vi "gRPC Client Test.vi"() -> ()   [LabVIEW 2024, in "pumploop_client.lvlib"]
uses:
  pumploop_client.lvlib
  controls/Controls--cluster.ctl
  controls/Sensors--cluster.ctl
  controls/SystemInfo--cluster.ctl
  controls/Valves--cluster.ctl
  <vilib>/gRPC/LabVIEW gRPC Library/Shared/grpcId.ctl
  controls/States.ctl
  controls/UI Queue Element.ctl
  RPC Messages/pumploop_GetSysInfRequest.ctl
  RPC Messages/pumploop_GetValveRequest.ctl
  RPC Messages/pumploop_GetControlRequest.ctl
  RPC Messages/pumploop_Controls.ctl
  RPC Messages/pumploop_Valves.ctl
  RPC Messages/pumploop_GetSensorRequest.ctl
  RPC Messages/pumploop_SystemInfo.ctl
  <vilib>/gRPC/LabVIEW gRPC Library/grpc-lvsupport-release.lvlib
panel:
  in  "Server Address":string="10.42.0.1:50051"
  in  "gRPC Disconnect":bool
  in  "gRPC Connect":bool
  in  "Stop":bool
  out "Error":errorcluster
  in  "Control Valves":T1
  out "Node Info":T2
  out "Sensors":T3 {"Pump Speed" scale=0.0..10.0; "Ambient Pressure" scale=0.5..1.5; "DUT Outlet Pressure" scale=0.0..2.0; "DUT Inlet Pressure" scale=0.0..10.0; "Flow" scale=0.0..100.0; "Sump Level" scale=0.0..100.0; "Tank Level" scale=0.0..100.0; "DUT Temp" scale=0.0..150.0; "Pump Temp" scale=0.0..150.0; "Tank Temp" scale=0.0..100.0; "Ambient Temp" scale=0.0..50.0}
  in  "Pump Control":T4
  in  "Stream":enum16{"Disabled", "Enabled"}(ring)
  in  "Subsystem":T5(ring)
  in  "Get/Set":enum16{"Get", "Set"}(ring)
  out "gRPC ID Out":u64
  # "192.168.0.141:50051"
  # "Open"
  # "Closed"
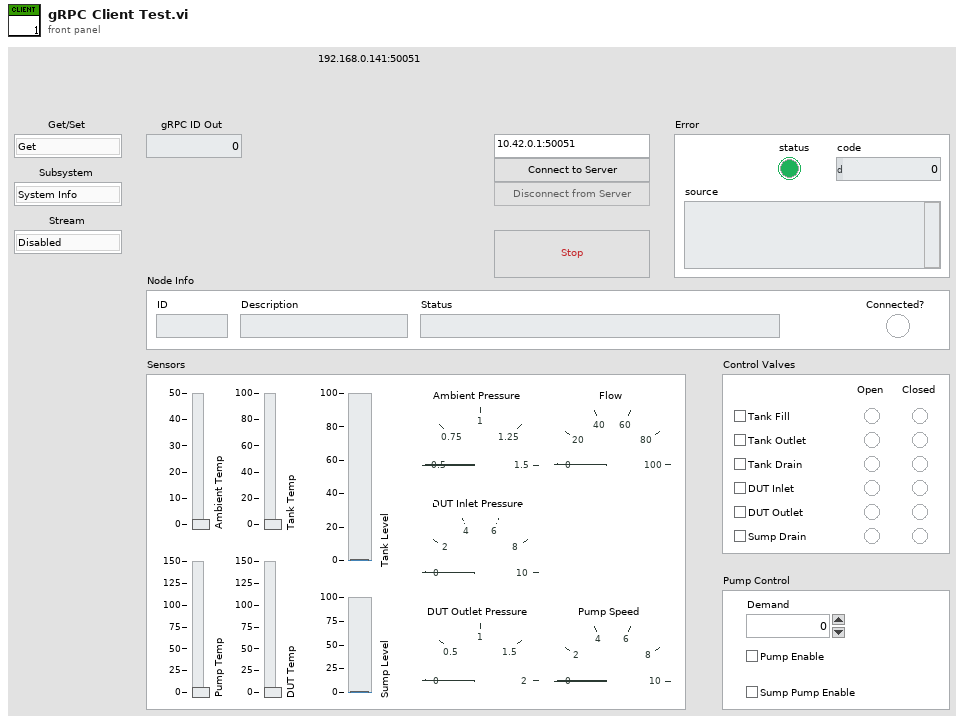
[diagram p1: front panel]
types:
  T1 = typedef "Valves--cluster.ctl" = cluster{"Tank Fill":bool, "Tank Outlet":bool, "Tank Drain":bool, "DUT Inlet":bool, "DUT Outlet":bool, "Sump Drain":bool, "Tank Fill Open":bool, "Tank Fill Closed":bool, "Tank Outlet Open":bool, "Tank Outlet Closed":bool, "Tank Drain Open":bool, "Tank Drain Closed":bool, "DUT Inlet Open":bool, "DUT Inlet Closed":bool, "DUT Outlet Open":bool, "DUT Outlet Closed":bool, "Sump Drain Open":bool, "Sump Drain Closed":bool}
  T2 = typedef "SystemInfo--cluster.ctl" = cluster{"Connected?":bool, "ID":string, "Description":string, "Status":string}
  T3 = typedef "Sensors--cluster.ctl" = cluster{"Tank Level":dbl, "Tank Temp":dbl, "Flow":dbl, "Pump Temp":dbl, "Pump Speed":dbl, "DUT Inlet Pressure":dbl, "DUT Outlet Pressure":dbl, "DUT Temp":dbl, "Sump Level":dbl, "Ambient Temp":dbl, "Ambient Pressure":dbl}
  T4 = typedef "Controls--cluster.ctl" = cluster{"Pump Enable":bool, "Demand":dbl, "Sump Pump Enable":bool}
  T5 = enum16{"System Info", "Valves", "Sensors", "Control"}
  T6 = typedef "UI Queue Element.ctl" = cluster{T7, variant}
  T7 = typedef "States.ctl" = enum16{"Initialise", "gRPC_Connect", "gRPC_Disconnect", "gRPC_Update-PumpCtrl", "gRPC_Update-ValveCtrl", "gRPC_ReadAll", "Update Settings", "Stop", "Quit"}
  T8 = cluster{"Node Info":T2, "Control Valves":T1, "Pump Control":T4, "Sensors":T3, "address":string}
  T9 = typedef "grpc-lvsupport-release.lvlib/grpcId.ctl" = u64
  T10 = typedef "pumploop_client.lvlib/pumploop_GetSysInfRequest.ctl" = cluster{"request":bool}
  T11 = typedef "pumploop_client.lvlib/pumploop_SystemInfo.ctl" = cluster{"nodeID":i32, "nodeDescription":string, "statusMsg":string}
  T12 = typedef "pumploop_client.lvlib/pumploop_GetValveRequest.ctl" = cluster{"request":bool}
  T13 = typedef "pumploop_client.lvlib/pumploop_Valves.ctl" = cluster{"tankFillIV":bool, "tankOutIV":bool, "tankDrainIV":bool, "dutInIV":bool, "dutOutIV":bool, "sumpDrainIV":bool}
  T14 = typedef "pumploop_client.lvlib/pumploop_GetSensorRequest.ctl" = cluster{"request":bool}
  T15 = typedef "pumploop_client.lvlib/pumploop_GetControlRequest.ctl" = cluster{"request":bool}
  T16 = typedef "pumploop_client.lvlib/pumploop_Controls.ctl" = cluster{"pumpEnable":bool, "pumpDemand":sgl, "sumppumpEnable":bool}
  T17 = typedef "pumploop_client.lvlib/pumploop_Sensors.ctl" = cluster{"tankLevel":sgl, "tankTemp":sgl, "dutFlow":sgl, "pumpTemp":sgl, "pumpSpeed":sgl, "dutPressIn":sgl, "dutPressOut":sgl, "dutTemp":sgl, "sumpLevel":sgl, "ambientTemp":sgl, "ambientPress":sgl}
  T18 = enum8{"Enabled", "Disabled", "Disabled and Grayed Out"}
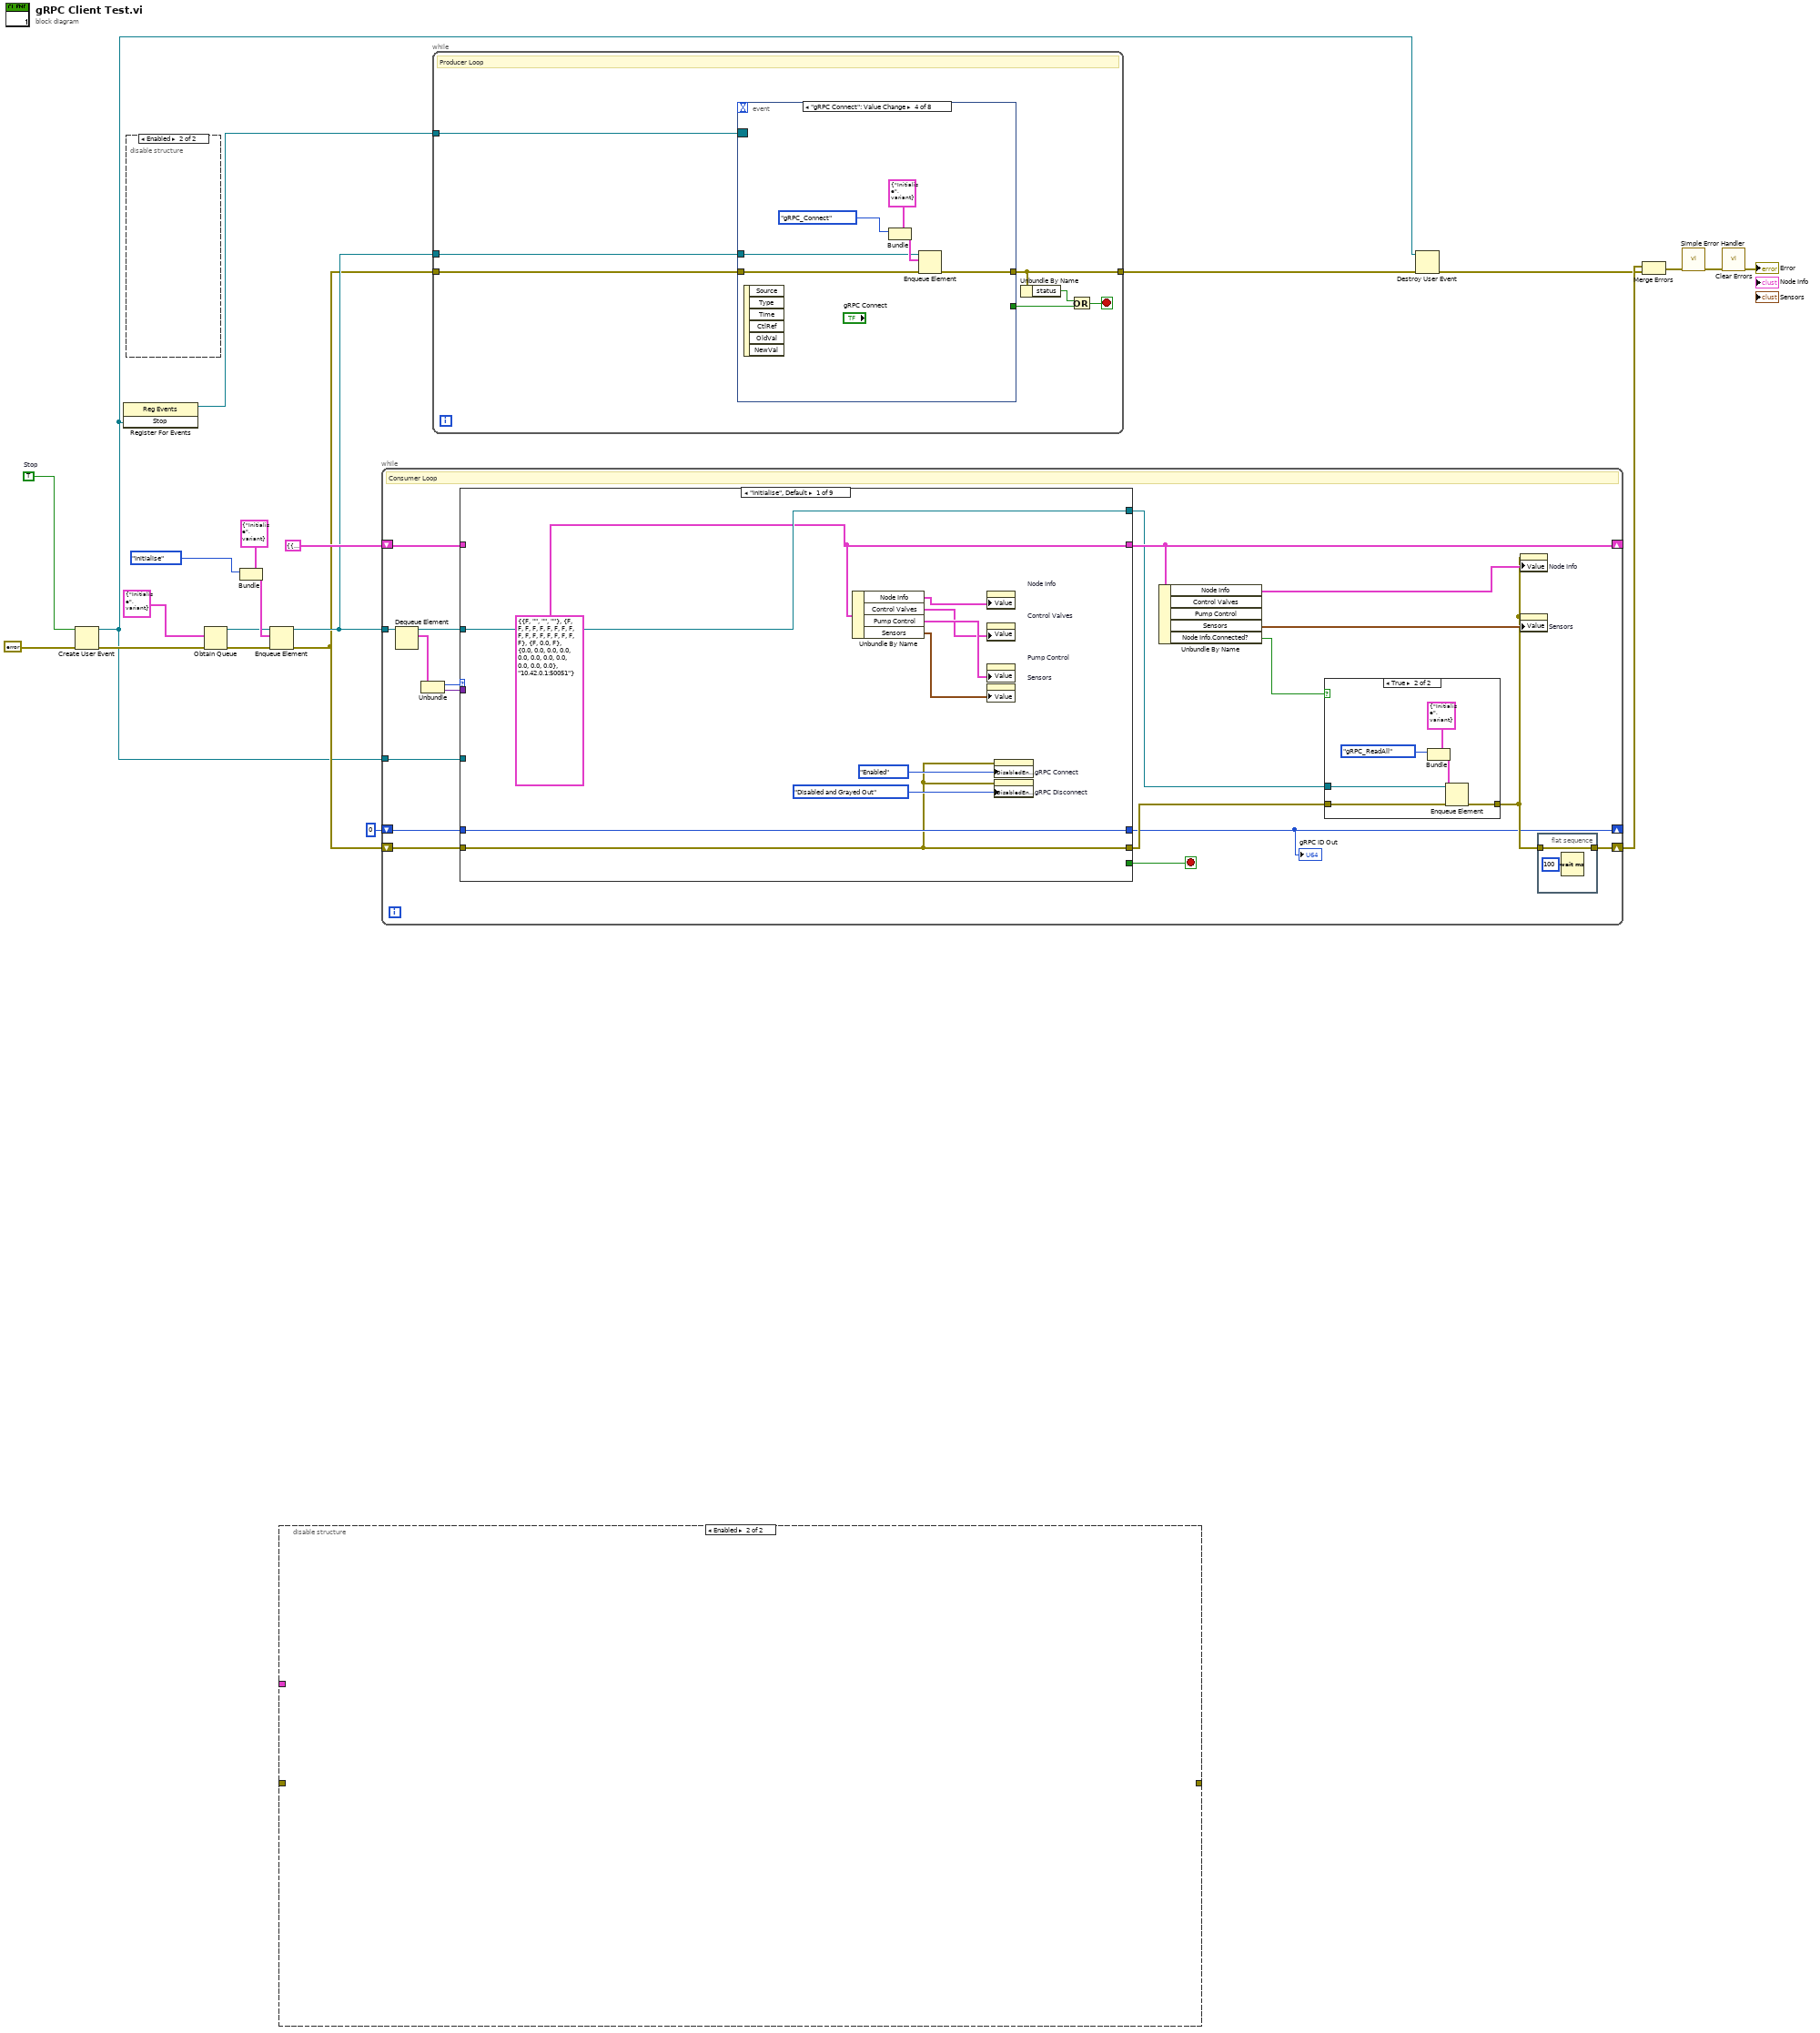
[diagram p0: block diagram]
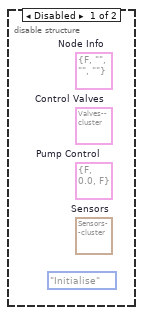
[diagram p2: hidden frame]
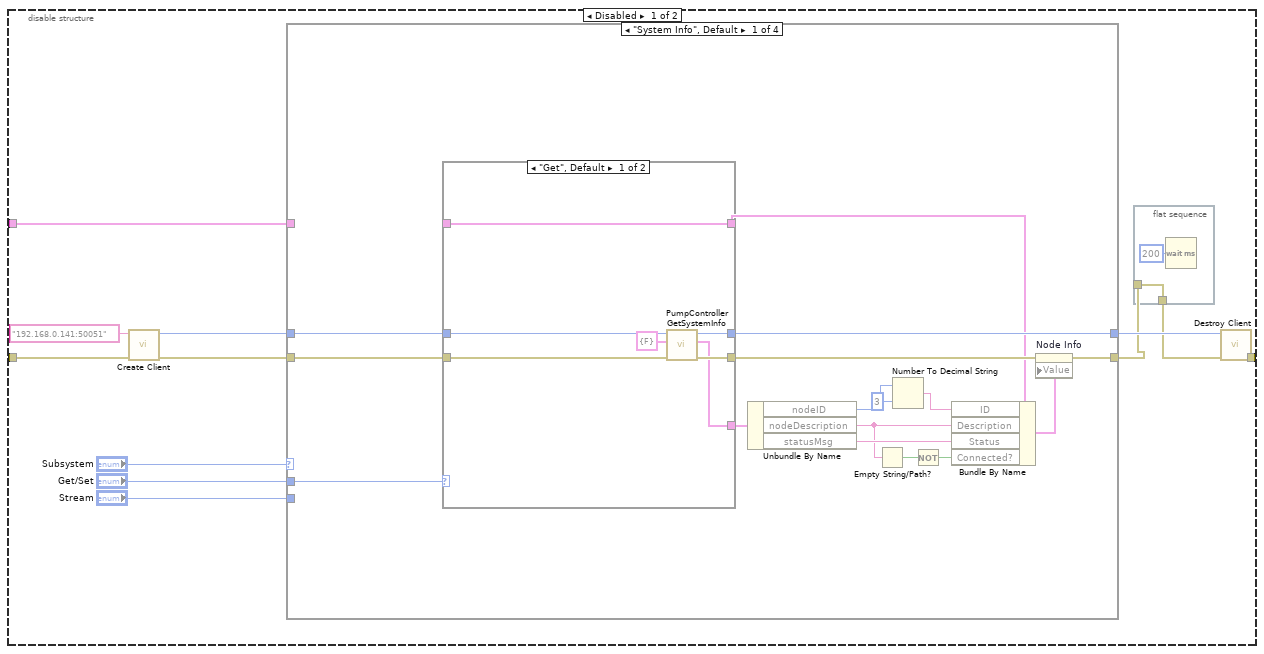
[diagram p3: hidden frame]
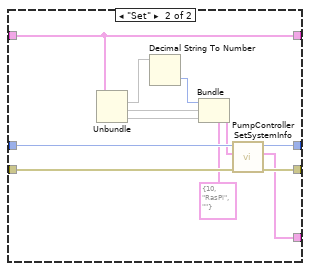
[diagram p4: hidden frame]
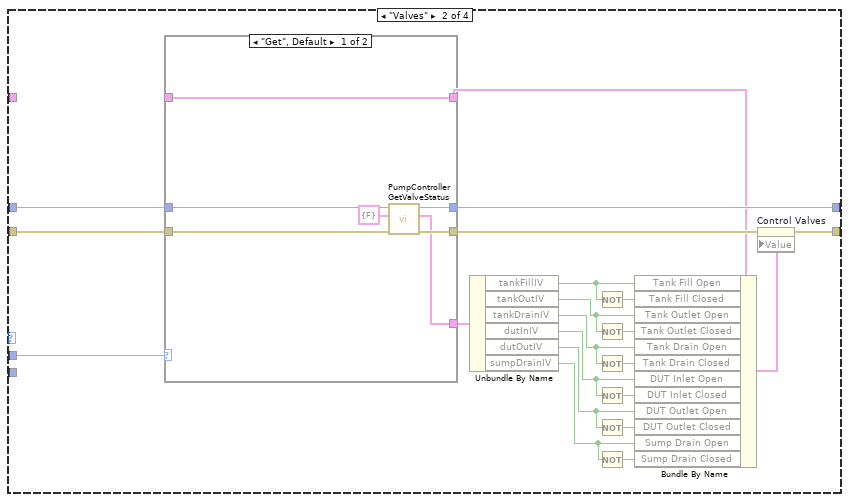
[diagram p5: hidden frame]
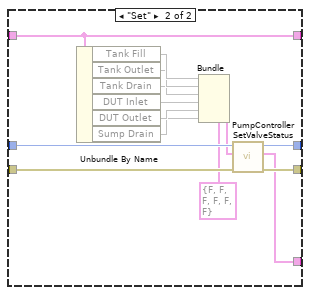
[diagram p6: hidden frame]
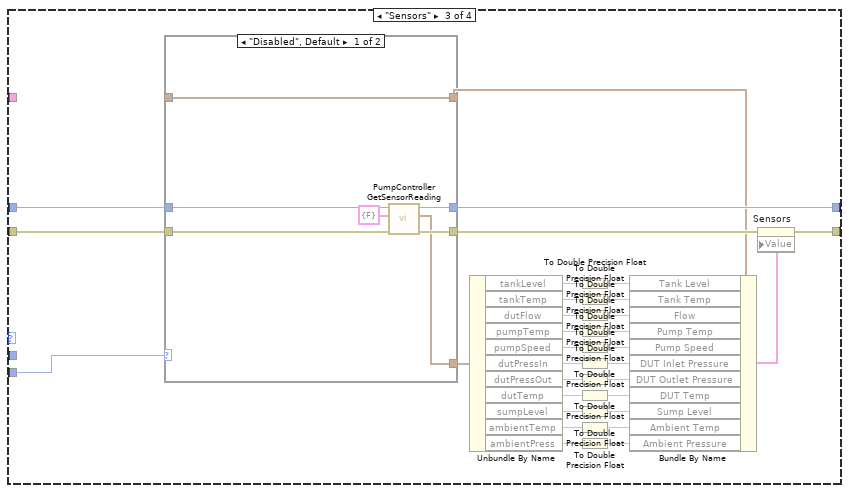
[diagram p7: hidden frame]
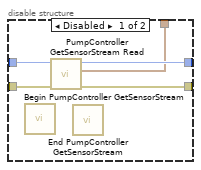
[diagram p9: hidden frame]
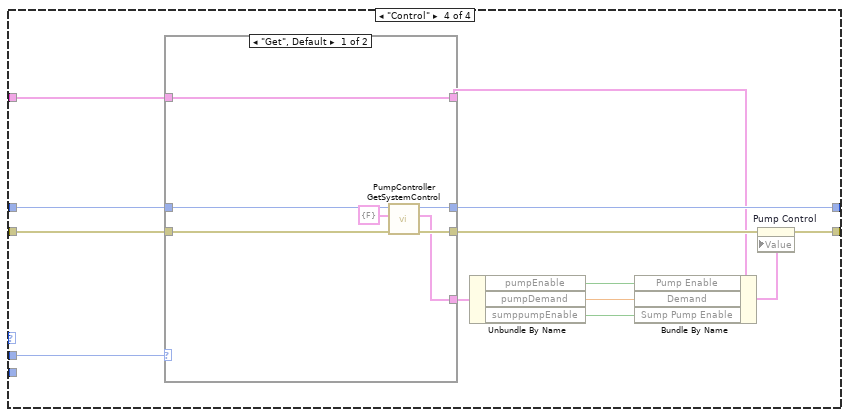
[diagram p10: hidden frame]
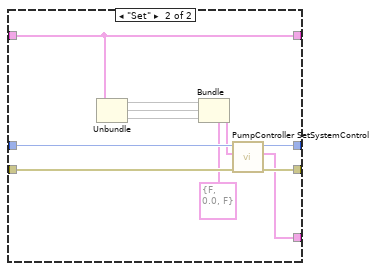
[diagram p11: hidden frame]
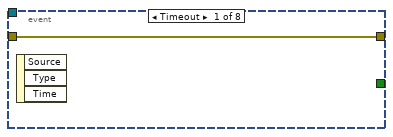
[diagram p12: hidden frame]
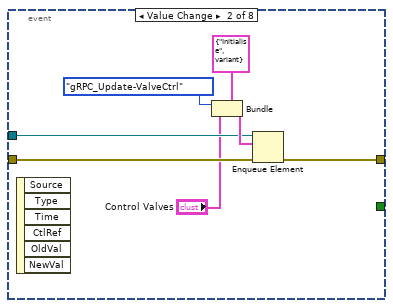
[diagram p13: hidden frame]
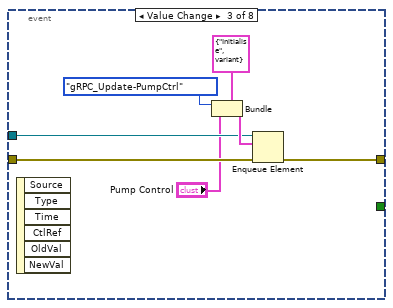
[diagram p14: hidden frame]
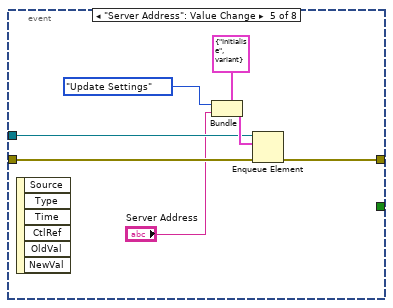
[diagram p15: hidden frame]
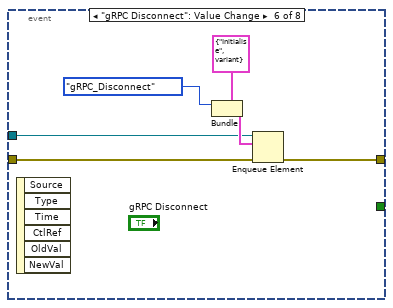
[diagram p16: hidden frame]
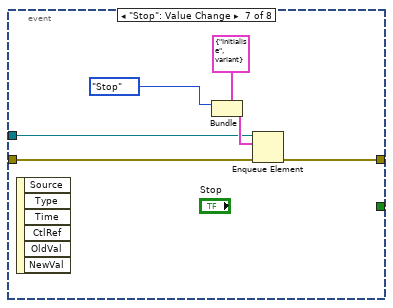
[diagram p17: hidden frame]
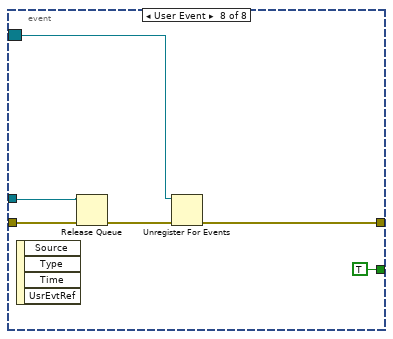
[diagram p18: hidden frame]
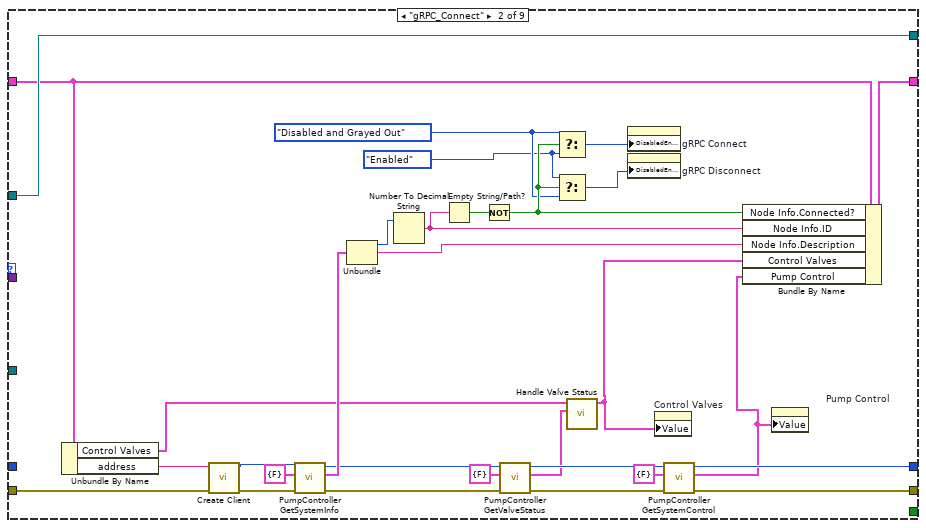
[diagram p20: hidden frame]
diagram:
  w7 = TRUE  # Stop
  n1 = Create User Event(user event datatype=w7, error in=errorcluster {"status"=FALSE, "code"=0, "source"=""}) -> (user event=w1:refnum<user-event>, error out=w5:errorcluster)
  n2 = register-events(w1) -> (reference out=w4:refnum<event-registration>)  [unwired: 2 in, 1 out]
  n3 = disable-structure shown="Enabled" {
    frame Disabled {
      (unwired) States."Initialise"
      (unwired) T3 {"Tank Level"=0.0, "Tank Temp"=0.0, "Flow"=0.0, "Pump Temp"=0.0, "Pump Speed"=0.0, "DUT Inlet Pressure"=0.0, "DUT Outlet Pressure"=0.0, "DUT Temp"=0.0, "Sump Level"=0.0, "Ambient Temp"=0.0, "Ambient Pressure"=0.0}  # Sensors
      (unwired) T4 {"Pump Enable"=FALSE, "Demand"=0.0, "Sump Pump Enable"=FALSE}  # Pump Control
      (unwired) T1 {"Tank Fill"=FALSE, "Tank Outlet"=FALSE, "Tank Drain"=FALSE, "DUT Inlet"=FALSE, "DUT Outlet"=FALSE, "Sump Drain"=FALSE, "Tank Fill Open"=FALSE, "Tank Fill Closed"=FALSE, "Tank Outlet Open"=FALSE, "Tank Outlet Closed"=FALSE, "Tank Drain Open"=FALSE, "Tank Drain Closed"=FALSE, "DUT Inlet Open"=FALSE, "DUT Inlet Closed"=FALSE, "DUT Outlet Open"=FALSE, "DUT Outlet Closed"=FALSE, "Sump Drain Open"=FALSE, "Sump Drain Closed"=FALSE}  # Control Valves
      (unwired) T2 {"Connected?"=FALSE, "ID"="", "Description"="", "Status"=""}  # Node Info
    }
    frame Enabled {
    }
  }
  n4 = Obtain Queue(element data type=T6 {enum."Initialise", variant}, error in (no error)=w5) -> (queue out=w12:refnum<queue>, error out=w11:errorcluster)  [unwired: 3 in, 1 out]
  n5 = Bundle(cluster=T6 {enum."Initialise", variant}, States."Initialise") -> (w15:T6)  [unwired: 1 in]
  n6 = Enqueue Element(queue=w12, element=w15, error in (no error)=w11) -> (queue out=w10:refnum<queue>, error out=w9:errorcluster)  [unwired: 1 in, 1 out]
  n7 = disable-structure shown="Enabled" {
    disable-tunnel: [w26 _] -> _
    disable-tunnel: _ -> [w23 _]
    disable-tunnel: _ -> [w22 _]
    frame Disabled {
      n8 = call "Create Client.vi"("error in"=w23, "address"="192.168.0.141:50051") -> ("error out"=w33:errorcluster, "gRPC ID Out"=w31:T9)  [unwired: 8 in]
      n9 = case shown="\"System Info\", Default" "Subsystem" {
        tunnel: w33 -> [w51 w91 w143 w174]
        tunnel: [w46 w87 w114 w166] -> w25
        tunnel: [w50 w90 w142 w173] -> w32
        tunnel: w31 -> [w49 w89 w141 w172]
        tunnel: "Get/Set" -> [w48 w88 _ w171]
        tunnel: "Stream" -> [_ _ w140 _]
        tunnel: w22 -> [_ _ _ w162]
        frame "System Info", Default {
          n10 = case shown="\"Get\", Default" w48 {
            tunnel: w51 -> [w58 w70]
            tunnel: [w56 w69] -> w47
            tunnel: [w55 w68] -> w50
            tunnel: w49 -> [w57 w67]
            tunnel: [w54 w66] -> w45
            tunnel: _ -> [w52 w64]
            tunnel: [w52 w64] -> w39
            frame "Get", Default {
              n11 = call "PumpController GetSystemInfo.vi"("error in"=w58, "Request Data"=T10 {"request"=FALSE}, "gRPC ID"=w57) -> ("error out"=w56:errorcluster, "Response Data"=w54:T11, "gRPC ID out"=w55:T9)  [unwired: 6 in]
            }
            frame "Set" {
              n12 = Unbundle(w64) -> ("ID"=w60, "Description"=w62, "Status"=w61)  [unwired: 1 out]
              n13 = Decimal String To Number(string=w60) -> (number=w59:i32)  [unwired: 2 in, 1 out]
              n14 = Bundle(cluster=T11 {"nodeID"=10, "nodeDescription"="RasPi", "statusMsg"=""} ("Node Info Request"), "nodeID"=w59, "nodeDescription"=w62, "statusMsg"=w61) -> (w63:T11)
              n15 = call "PumpController SetSystemInfo.vi"("error in"=w70, "Request Data"=w63, "gRPC ID"=w67) -> ("error out"=w69:errorcluster, "Response Data"=w66:T11, "gRPC ID out"=w68:T9)  [unwired: 6 in]
            }
          }
          n16 = Unbundle By Name(w45) -> ("nodeID"=w42:i32, "nodeDescription"=w38:string, "statusMsg"=w43:string)
          n17 = Empty String/Path?(string/path=w38) -> (empty?=w37:bool)
          n18 = Number To Decimal String(number=w42, width (-)=i16 3) -> (decimal integer string=w41:string)
          n19 = Not(x=w37) -> (.not. x?=w36:bool)
          n20 = Bundle By Name(cluster=w39, "ID"=w41, "Description"=w38, "Status"=w43, "Connected?"=w36) -> (w44:cluster{})
          n21 = property on="Node Info" class="Clust (strict)"(error in=w47, "Value"=w44) -> (error out=w46:errorcluster)  [unwired: 1 in, 1 out]
        }
        frame "Valves" {
          n22 = case shown="\"Get\", Default" w88 {
            tunnel: w91 -> [w97 w111]
            tunnel: [w96 w109] -> w86
            tunnel: [w95 w110] -> w90
            tunnel: w89 -> [w98 w112]
            tunnel: [w94 w108] -> w85
            tunnel: _ -> [w92 w99]
            tunnel: [w92 w99] -> w71
            frame "Get", Default {
              n23 = call "PumpController GetValveStatus.vi"("error in"=w97, "Request Data"=T12 {"request"=FALSE}, "gRPC ID"=w98) -> ("error out"=w96:errorcluster, "Response Data"=w94:T13, "gRPC ID out"=w95:T9)  [unwired: 6 in]
            }
            frame "Set" {
              n24 = Unbundle By Name(w99) -> ("Tank Fill"=w106, "Tank Outlet"=w105, "Tank Drain"=w104, "DUT Inlet"=w103, "DUT Outlet"=w102, "Sump Drain"=w101)
              n25 = Bundle(cluster=T13 {"tankFillIV"=FALSE, "tankOutIV"=FALSE, "tankDrainIV"=FALSE, "dutInIV"=FALSE, "dutOutIV"=FALSE, "sumpDrainIV"=FALSE} ("Valve Control Request"), "tankFillIV"=w106, "tankOutIV"=w105, "tankDrainIV"=w104, "dutInIV"=w103, "dutOutIV"=w102, "sumpDrainIV"=w101) -> (w100:T13)
              n26 = call "PumpController SetValveStatus.vi"("error in"=w111, "Request Data"=w100, "gRPC ID"=w112) -> ("error out"=w109:errorcluster, "Response Data"=w108:T13, "gRPC ID out"=w110:T9)  [unwired: 6 in]
            }
          }
          n27 = Unbundle By Name(w85) -> ("tankFillIV"=w76:bool, "tankOutIV"=w75:bool, "tankDrainIV"=w77:bool, "dutInIV"=w74:bool, "dutOutIV"=w73:bool, "sumpDrainIV"=w72:bool)
          n28 = Not(x=w76) -> (.not. x?=w83:bool)
          n29 = Not(x=w75) -> (.not. x?=w82:bool)
          n30 = Not(x=w77) -> (.not. x?=w81:bool)
          n31 = Not(x=w74) -> (.not. x?=w80:bool)
          n32 = Not(x=w73) -> (.not. x?=w79:bool)
          n33 = Not(x=w72) -> (.not. x?=w78:bool)
          n34 = Bundle By Name(cluster=w71, "Tank Fill Open"=w76, "Tank Fill Closed"=w83, "Tank Outlet Open"=w75, "Tank Outlet Closed"=w82, "Tank Drain Open"=w77, "Tank Drain Closed"=w81, "DUT Inlet Open"=w74, "DUT Inlet Closed"=w80, "DUT Outlet Open"=w73, "DUT Outlet Closed"=w79, "Sump Drain Open"=w72, "Sump Drain Closed"=w78) -> (w84:cluster{})
          n35 = property on="Control Valves" class="Clust (strict)"(error in=w86, "Value"=w84) -> (error out=w87:errorcluster)  [unwired: 1 in, 1 out]
        }
        frame "Sensors" {
          n36 = case shown="\"Disabled\", Default" w140 {
            tunnel: w143 -> [w147 w153]
            tunnel: [w149 w156] -> w115
            tunnel: [w150 w155] -> w142
            tunnel: w141 -> [w148 w154]
            tunnel: [w145 w152] -> w139
            tunnel: [w144 w151] -> w113
            tunnel: _ -> [w144 w151]
            frame "Disabled", Default {
              n37 = call "PumpController GetSensorReading.vi"("error in"=w147, "Request Data"=T14 {"request"=FALSE}, "gRPC ID"=w148) -> ("error out"=w149:errorcluster, "Response Data"=w145:T17, "gRPC ID out"=w150:T9)  [unwired: 6 in]
            }
            frame "Enabled" {
              n38 = disable-structure shown="Enabled" {
                disable-tunnel: [w161 _] -> w156
                disable-tunnel: [w160 _] -> w155
                disable-tunnel: w154 -> [w159 _]
                disable-tunnel: w153 -> [w158 _]
                disable-tunnel: [w157 _] -> w152
                frame Disabled {
                  n39 = call "Begin PumpController GetSensorStream.vi"() -> ()  [unwired: 9 in, 3 out]
                  n40 = call "PumpController GetSensorStream Read.vi"("error in"=w158, "Call ID in"=w159) -> ("error out"=w161:errorcluster, "Response Data"=w157:T17, "Call ID"=w160:T9)  [unwired: 6 in, 1 out]
                  n41 = call "End PumpController GetSensorStream.vi"() -> ()  [unwired: 10 in, 2 out]
                }
                frame Enabled {
                }
              }
            }
          }
          n42 = Unbundle By Name(w139) -> ("tankLevel"=w138:sgl, "tankTemp"=w137:sgl, "dutFlow"=w136:sgl, "pumpTemp"=w134:sgl, "pumpSpeed"=w133:sgl, "dutPressIn"=w135:sgl, "dutPressOut"=w132:sgl, "dutTemp"=w131:sgl, "sumpLevel"=w130:sgl, "ambientTemp"=w129:sgl, "ambientPress"=w128:sgl)
          n43 = To Double Precision Float(number=w138) -> (double precision float=w127:dbl)
          n44 = To Double Precision Float(number=w137) -> (double precision float=w126:dbl)
          n45 = To Double Precision Float(number=w136) -> (double precision float=w125:dbl)
          n46 = To Double Precision Float(number=w134) -> (double precision float=w124:dbl)
          n47 = To Double Precision Float(number=w133) -> (double precision float=w123:dbl)
          n48 = To Double Precision Float(number=w135) -> (double precision float=w122:dbl)
          n49 = To Double Precision Float(number=w132) -> (double precision float=w121:dbl)
          n50 = To Double Precision Float(number=w131) -> (double precision float=w120:dbl)
          n51 = To Double Precision Float(number=w130) -> (double precision float=w119:dbl)
          n52 = To Double Precision Float(number=w129) -> (double precision float=w118:dbl)
          n53 = To Double Precision Float(number=w128) -> (double precision float=w117:dbl)
          n54 = Bundle By Name(cluster=w113, "Tank Level"=w127, "Tank Temp"=w126, "Flow"=w125, "Pump Temp"=w124, "Pump Speed"=w123, "DUT Inlet Pressure"=w122, "DUT Outlet Pressure"=w121, "DUT Temp"=w120, "Sump Level"=w119, "Ambient Temp"=w118, "Ambient Pressure"=w117) -> (w116:cluster{})
          n55 = property on="Sensors" class="Clust (strict)"(error in=w115, "Value"=w116) -> (error out=w114:errorcluster)  [unwired: 1 in, 1 out]
        }
        frame "Control" {
          n56 = case shown="\"Get\", Default" w171 {
            tunnel: w174 -> [w180 w191]
            tunnel: [w178 w189] -> w165
            tunnel: [w179 w190] -> w173
            tunnel: w172 -> [w181 w192]
            tunnel: [w177 w188] -> w170
            tunnel: w162 -> [w175 w183]
            tunnel: [w175 w183] -> w163
            frame "Get", Default {
              n57 = call "PumpController GetSystemControl.vi"("error in"=w180, "Request Data"=T15 {"request"=FALSE}, "gRPC ID"=w181) -> ("error out"=w178:errorcluster, "Response Data"=w177:T16, "gRPC ID out"=w179:T9)  [unwired: 6 in]
            }
            frame "Set" {
              n58 = Unbundle(w183) -> ("Pump Enable"=w186, "Demand"=w187, "Sump Pump Enable"=w182)
              n59 = Bundle(cluster=T16 {"pumpEnable"=FALSE, "pumpDemand"=0.0, "sumppumpEnable"=FALSE} ("System Control Request"), "pumpEnable"=w186, "pumpDemand"=w187, "sumppumpEnable"=w182) -> (w185:T16)
              n60 = call "PumpController SetSystemControl.vi"("error in"=w191, "Request Data"=w185, "gRPC ID"=w192) -> ("error out"=w189:errorcluster, "Response Data"=w188:T16, "gRPC ID out"=w190:T9)  [unwired: 6 in]
            }
          }
          n61 = Unbundle By Name(w170) -> ("pumpEnable"=w169:bool, "pumpDemand"=w168:sgl, "sumppumpEnable"=w167:bool)
          n62 = Bundle By Name(cluster=w163, "Pump Enable"=w169, "Demand"=w168, "Sump Pump Enable"=w167) -> (w164:cluster{})
          n63 = property on="Pump Control" class="Clust (strict)"(error in=w165, "Value"=w164) -> (error out=w166:errorcluster)  [unwired: 1 in, 1 out]
        }
      }
      n64 = flat-sequence {
        tunnel: w25 -> [w35]
        tunnel: [w35] -> w24
        frame #0 {
          n65 = Wait (ms)(milliseconds to wait=u32 200) -> ()  [unwired: 1 out]
        }
      }
      n66 = call "Destroy Client.vi"("error in"=w24, "gRPC ID"=w32) -> ("error out"=w26:errorcluster)  [unwired: 9 in]
    }
    frame Enabled {
    }
  }
  n67 = while {
    shift-right: [w197] -> w18
    shift-left: w9 -> [w211]
    shift-right: [w194] -> _
    shift-left: T9 0 ("gRPC ID Out") -> [w210]
    tunnel: w10 -> [w209]
    shift-right: [w203] -> _
    shift-left: T8 {"Node Info"={"Connected?"=FALSE, "ID"="", "Description"="", "Status"=""}, "Control Valves"={"Tank Fill"=FALSE, "Tank Outlet"=FALSE, "Tank Drain"=FALSE, "DUT Inlet"=FALSE, "DUT Outlet"=FALSE, "Sump Drain"=FALSE, "Tank Fill Open"=FALSE, "Tank Fill Closed"=FALSE, "Tank Outlet Open"=FALSE, "Tank Outlet Closed"=FALSE, "Tank Drain Open"=FALSE, "Tank Drain Closed"=FALSE, "DUT Inlet Open"=FALSE, "DUT Inlet Closed"=FALSE, "DUT Outlet Open"=FALSE, "DUT Outlet Closed"=FALSE, "Sump Drain Open"=FALSE, "Sump Drain Closed"=FALSE}, "Pump Control"={"Pump Enable"=FALSE, "Demand"=0.0, "Sump Pump Enable"=FALSE}, "Sensors"={"Tank Level"=0.0, "Tank Temp"=0.0, "Flow"=0.0, "Pump Temp"=0.0, "Pump Speed"=0.0, "DUT Inlet Pressure"=0.0, "DUT Outlet Pressure"=0.0, "DUT Temp"=0.0, "Sump Level"=0.0, "Ambient Temp"=0.0, "Ambient Pressure"=0.0}, "address"="192.168.0.141:50051"} -> [w204]
    tunnel: w1 -> [w193]
    stop <- w200 stop-if-true
    # "Consumer Loop"
    n68 = Dequeue Element(queue=w209) -> (queue out=w206:refnum<queue>, element=w208:T6)  [unwired: 2 in, 2 out]
    n69 = Unbundle(w208) -> (w207:T7, w205:variant)
    n70 = case shown="\"Initialise\", Default" w207 {
      tunnel: w211 -> [w226 w260 w271 w277 w295 w299 w309 w339 w375]
      tunnel: [w226 w240 w263 w276 w287 w298 w312 w336 w374] -> w196
      tunnel: [w230 w237 T9 0 ("gRPC ID Out") w284 w286 w304 w311 w335 w373] -> w194
      tunnel: w210 -> [w230 _ w270 w284 w286 w304 w313 w337 w372]
      tunnel: w206 -> [w229 w259 w268 w283 w290 w301 w307 w334 w370]
      tunnel: w205 -> [_ _ _ w280 _ _ w310 w340 _]
      tunnel: w204 -> [_ w253 w261 w282 w285 w303 w306 w332 w369]
      tunnel: [w221 w252 w267 w281 w285 w303 w308 w338 w371] -> w203
      tunnel: [_ _ _ _ _ TRUE _ _ _] -> w200
      tunnel: [w229 w259 w268 w283 w290 w301 w307 w334 w370] -> w199
      tunnel: w193 -> [_ _ _ _ _ w300 _ _ _]
      frame "Initialise", Default {
        w221 = T8 {"Node Info"={"Connected?"=FALSE, "ID"="", "Description"="", "Status"=""}, "Control Valves"={"Tank Fill"=FALSE, "Tank Outlet"=FALSE, "Tank Drain"=FALSE, "DUT Inlet"=FALSE, "DUT Outlet"=FALSE, "Sump Drain"=FALSE, "Tank Fill Open"=FALSE, "Tank Fill Closed"=FALSE, "Tank Outlet Open"=FALSE, "Tank Outlet Closed"=FALSE, "Tank Drain Open"=FALSE, "Tank Drain Closed"=FALSE, "DUT Inlet Open"=FALSE, "DUT Inlet Closed"=FALSE, "DUT Outlet Open"=FALSE, "DUT Outlet Closed"=FALSE, "Sump Drain Open"=FALSE, "Sump Drain Closed"=FALSE}, "Pump Control"={"Pump Enable"=FALSE, "Demand"=0.0, "Sump Pump Enable"=FALSE}, "Sensors"={"Tank Level"=0.0, "Tank Temp"=0.0, "Flow"=0.0, "Pump Temp"=0.0, "Pump Speed"=0.0, "DUT Inlet Pressure"=0.0, "DUT Outlet Pressure"=0.0, "DUT Temp"=0.0, "Sump Level"=0.0, "Ambient Temp"=0.0, "Ambient Pressure"=0.0}, "address"="10.42.0.1:50051"}
        n71 = Unbundle By Name(w221) -> ("Node Info"=w223:T2, "Control Valves"=w222:T1, "Pump Control"=w224:T4, "Sensors"=w225:T3)
        n72 = property on="Node Info" class="Clust (strict)"("Value"=w223) -> ()  [unwired: 2 in, 2 out]
        n73 = property on="Control Valves" class="Clust (strict)"("Value"=w222) -> ()  [unwired: 2 in, 2 out]
        n74 = property on="Pump Control" class="Clust (strict)"("Value"=w224) -> ()  [unwired: 2 in, 2 out]
        n75 = property on="Sensors" class="Clust (strict)"("Value"=w225) -> ()  [unwired: 2 in, 2 out]
        n76 = property on="gRPC Connect" class="Bool (strict)"(error in=w226, "DisabledEnum"=T18."Enabled" ("Disabled")) -> ()  [unwired: 1 in, 2 out]
        n77 = property on="gRPC Disconnect" class="Bool (strict)"(error in=w226, "DisabledEnum"=T18."Disabled and Grayed Out" ("Disabled")) -> ()  [unwired: 1 in, 2 out]
      }
      frame "gRPC_Connect" {
        w245 = T18."Enabled" ("Disabled")
        w246 = T18."Disabled and Grayed Out" ("Disabled")
        n78 = Unbundle By Name(w253) -> ("Control Valves"=w233:T1, "address"=w258:string)
        n79 = call "Create Client.vi"("error in"=w260, "address"=w258) -> ("error out"=w250:errorcluster, "gRPC ID Out"=w249:T9)  [unwired: 8 in]
        n80 = call "PumpController GetSystemInfo.vi"("error in"=w250, "Request Data"=T10 {"request"=FALSE}, "gRPC ID"=w249) -> ("error out"=w241:errorcluster, "Response Data"=w254:T11, "gRPC ID out"=w239:T9)  [unwired: 6 in]
        n81 = Unbundle(w254) -> ("nodeID"=w257:i32, "nodeDescription"=w256:string)  [unwired: 1 out]
        n82 = Number To Decimal String(number=w257) -> (decimal integer string=w255:string)  [unwired: 1 in]
        n83 = Empty String/Path?(string/path=w255) -> (empty?=w248:bool)
        n84 = Not(x=w248) -> (.not. x?=w247:bool)
        n85 = call "PumpController GetValveStatus.vi"("error in"=w241, "Request Data"=T12 {"request"=FALSE}, "gRPC ID"=w239) -> ("error out"=w242:errorcluster, "Response Data"=w234:T13, "gRPC ID out"=w238:T9)  [unwired: 6 in]
        n86 = Select(t=w246, s=w247, f=w245) -> (s? t:f=w244:T18)
        n87 = Select(t=w245, s=w247, f=w246) -> (s? t:f=w243:T18)
        n88 = call "Handle Valve Status.vi"("Response Data"=w234, "Control Valves in"=w233) -> ("Control Valves out"=w232:T1)  [unwired: 9 in]
        n89 = property on="gRPC Connect" class="Bool (strict)"("DisabledEnum"=w244) -> ()  [unwired: 2 in, 2 out]
        n90 = property on="gRPC Disconnect" class="Bool (strict)"("DisabledEnum"=w243) -> ()  [unwired: 2 in, 2 out]
        n91 = property on="Control Valves" class="Clust (strict)"("Value"=w232) -> ()  [unwired: 2 in, 2 out]
        n92 = call "PumpController GetSystemControl.vi"("error in"=w242, "Request Data"=T15 {"request"=FALSE}, "gRPC ID"=w238) -> ("error out"=w240:errorcluster, "Response Data"=w231:T16, "gRPC ID out"=w237:T9)  [unwired: 6 in]
        n93 = Bundle By Name(cluster=w253, "Node Info.Connected?"=w247, "Node Info.ID"=w255, "Node Info.Description"=w256, "Control Valves"=w232, "Pump Control"=w231) -> (w252:T8)
        n94 = property on="Pump Control" class="Clust (strict)"("Value"=w231) -> ()  [unwired: 2 in, 2 out]
      }
      frame "gRPC_Disconnect" {
        n95 = Unbundle By Name(w261) -> ("Node Info.Connected?"=w262:bool)
        n96 = case shown="False" w262 {
          tunnel: w271 -> [w272 w275]
          tunnel: w270 -> [_ w274]
          tunnel: [w272 w273] -> w263
          frame False {
          }
          frame True {
            n97 = call "Destroy Client.vi"("error in"=w275, "gRPC ID"=w274) -> ("error out"=w273:errorcluster)  [unwired: 9 in]
          }
        }
        n98 = Bundle By Name(cluster=w261, "Node Info.Connected?"=FALSE) -> (w267:T8)
        n99 = property on="gRPC Connect" class="Bool (strict)"(error in=w263, "DisabledEnum"=T18."Enabled" ("Disabled")) -> ()  [unwired: 1 in, 2 out]
        n100 = property on="gRPC Disconnect" class="Bool (strict)"(error in=w263, "DisabledEnum"=T18."Disabled and Grayed Out" ("Disabled")) -> ()  [unwired: 1 in, 2 out]
      }
      frame "Update Settings" {
        n101 = Variant To Data(error in=w277, type="", Variant=w280) -> (data=w278:string, error out=w276:errorcluster)
        n102 = Bundle By Name(cluster=w282, "address"=w278) -> (w281:T8)
      }
      frame "Stop" {
        w288 = T6 {enum."Initialise", variant}
        n103 = Bundle(cluster=w288, States."gRPC_Disconnect") -> (w294:T6)  [unwired: 1 in]
        n104 = Enqueue Element(queue=w290, element=w294, error in (no error)=w295) -> (queue out=w291:refnum<queue>, error out=w292:errorcluster)  [unwired: 1 in, 1 out]
        n105 = Bundle(cluster=w288, States."Quit") -> (w289:T6)  [unwired: 1 in]
        n106 = Enqueue Element(queue=w291, element=w289, error in (no error)=w292) -> (error out=w287:errorcluster)  [unwired: 1 in, 2 out]
      }
      frame "Quit" {
        n107 = Generate User Event(user event=w300, event data cluster=TRUE ("event data"), error in=w299) -> (error out=w298:errorcluster)  [unwired: 1 in, 1 out]
      }
      frame "gRPC_Update-PumpCtrl" {
        n108 = Unbundle By Name(w306) -> ("Node Info.Connected?"=w305:bool)
        n109 = case shown="False" w305 {
          tunnel: w313 -> [w315 w326]
          tunnel: [w314 w325] -> w312
          tunnel: [w315 w324] -> w311
          tunnel: w310 -> [_ w323]
          tunnel: w309 -> [w314 w322]
          tunnel: w306 -> [w316 w319]
          tunnel: [w316 w317] -> w308
          frame False {
          }
          frame True {
            n110 = Variant To Data(error in=w322, type=T4 {"Pump Enable"=FALSE, "Demand"=0.0, "Sump Pump Enable"=FALSE} ("Pump Control"), Variant=w323) -> (data=w318:T4, error out=w321:errorcluster)
            n111 = Unbundle(w318) -> ("Pump Enable"=w328:bool, "Demand"=w327:dbl, "Sump Pump Enable"=w331:bool)
            n112 = Bundle(cluster=T16 {"pumpEnable"=FALSE, "pumpDemand"=0.0, "sumppumpEnable"=FALSE} ("System Control Request"), "pumpEnable"=w328, "pumpDemand"=w327, "sumppumpEnable"=w331) -> (w329:T16)
            n113 = Bundle By Name(cluster=w319, "Pump Control"=w318) -> (w317:T8)
            n114 = call "PumpController SetSystemControl.vi"("error in"=w321, "Request Data"=w329, "gRPC ID"=w326) -> ("error out"=w325:errorcluster, "gRPC ID out"=w324:T9)  [unwired: 6 in, 1 out]
          }
        }
      }
      frame "gRPC_Update-ValveCtrl" {
        n115 = Unbundle By Name(w332) -> ("Node Info.Connected?"=w333:bool)
        n116 = case shown="True" w333 {
          tunnel: w340 -> [_ w365]
          tunnel: w339 -> [w341 w364]
          tunnel: w332 -> [w343 w362]
          tunnel: [w343 w345] -> w338
          tunnel: w337 -> [w342 w355]
          tunnel: [w341 w349] -> w336
          tunnel: [w342 w348] -> w335
          frame False {
          }
          frame True {
            n117 = Variant To Data(error in=w364, type=T1 {"Tank Fill"=FALSE, "Tank Outlet"=FALSE, "Tank Drain"=FALSE, "DUT Inlet"=FALSE, "DUT Outlet"=FALSE, "Sump Drain"=FALSE, "Tank Fill Open"=FALSE, "Tank Fill Closed"=FALSE, "Tank Outlet Open"=FALSE, "Tank Outlet Closed"=FALSE, "Tank Drain Open"=FALSE, "Tank Drain Closed"=FALSE, "DUT Inlet Open"=FALSE, "DUT Inlet Closed"=FALSE, "DUT Outlet Open"=FALSE, "DUT Outlet Closed"=FALSE, "Sump Drain Open"=FALSE, "Sump Drain Closed"=FALSE} ("Control Valves"), Variant=w365) -> (data=w361:T1, error out=w354:errorcluster)
            n118 = Unbundle By Name(w361) -> ("Tank Fill"=w366:bool, "Tank Outlet"=w359:bool, "Tank Drain"=w367:bool, "DUT Inlet"=w358:bool, "DUT Outlet"=w357:bool, "Sump Drain"=w356:bool)
            n119 = Bundle By Name(cluster=w362, "Control Valves"=w361) -> (w345:T8)
            n120 = Bundle By Name(cluster=T13 {"tankFillIV"=FALSE, "tankOutIV"=FALSE, "tankDrainIV"=FALSE, "dutInIV"=FALSE, "dutOutIV"=FALSE, "sumpDrainIV"=FALSE} ("Valve Control Request"), "tankFillIV"=w366, "tankOutIV"=w359, "tankDrainIV"=w367, "dutInIV"=w358, "dutOutIV"=w357, "sumpDrainIV"=w356) -> (w353:T13)
            n121 = call "PumpController SetValveStatus.vi"("error in"=w354, "Request Data"=w353, "gRPC ID"=w355) -> ("error out"=w351:errorcluster, "gRPC ID out"=w350:T9)  [unwired: 6 in, 1 out]
            n122 = Unbundle By Name(w345) -> ("Control Valves"=w344:T1)
            n123 = call "PumpController GetValveStatus.vi"("error in"=w351, "Request Data"=T12 {"request"=FALSE}, "gRPC ID"=w350) -> ("error out"=w349:errorcluster, "Response Data"=w352:T13, "gRPC ID out"=w348:T9)  [unwired: 6 in]
            n124 = call "Handle Valve Status.vi"("Response Data"=w352, "Control Valves in"=w344) -> ("Control Valves out"=w346:T1)  [unwired: 9 in]
            n125 = property on="Control Valves" class="Clust (strict)"("Value"=w346) -> ()  [unwired: 2 in, 2 out]
          }
        }
      }
      frame "gRPC_ReadAll" {
        n126 = Unbundle By Name(w369) -> ("Node Info.Connected?"=w368:bool)
        n127 = case shown="True" w368 {
          tunnel: w375 -> [w378 w397]
          tunnel: [w378 w381] -> w374
          tunnel: [w377 w382] -> w373
          tunnel: w372 -> [w377 w396]
          tunnel: w369 -> [w376 w390]
          tunnel: [w376 w388] -> w371
          frame False {
          }
          frame True {
            n128 = call "PumpController GetSystemInfo.vi"("error in"=w397, "Request Data"=T10 {"request"=FALSE}, "gRPC ID"=w396) -> ("error out"=w379:errorcluster, "Response Data"=w395:T11, "gRPC ID out"=w380:T9)  [unwired: 6 in]
            n129 = Unbundle(w395) -> ("nodeID"=w394:i32, "statusMsg"=w393:string)  [unwired: 1 out]
            n130 = Unbundle By Name(w390) -> ("Node Info"=w389:T2)  [unwired: 1 out]
            n131 = Number To Decimal String(number=w394) -> (decimal integer string=w392:string)  [unwired: 1 in]
            n132 = Empty String/Path?(string/path=w392) -> (empty?=w384:bool)
            n133 = Not(x=w384) -> (.not. x?=w383:bool)
            n134 = Bundle By Name(cluster=w389, "Connected?"=w383, "Status"=w393) -> (w391:T2)
            n135 = call "PumpController GetSensorReading.vi"("error in"=w379, "Request Data"=T14 {"request"=FALSE}, "gRPC ID"=w380) -> ("error out"=w381:errorcluster, "Response Data"=w387:T17, "gRPC ID out"=w382:T9)  [unwired: 6 in]
            n136 = Bundle By Name(cluster=w390, "Node Info"=w391, "Sensors"=w387) -> (w388:T8)
          }
        }
      }
    }
    "gRPC ID Out" <- w194
    n137 = Unbundle By Name(w203) -> ("Node Info"=w202:T2, "Sensors"=w201:T3, "Node Info.Connected?"=w195:bool)  [unwired: 2 out]
    n138 = case shown="True" w195 {
      tunnel: w199 -> [_ w215]
      tunnel: [w212 w214] -> w198
      tunnel: w196 -> [w212 w213]
      frame False {
      }
      frame True {
        n139 = Bundle(cluster=T6 {enum."Initialise", variant}, States."gRPC_ReadAll") -> (w217:T6)  [unwired: 1 in]
        n140 = Enqueue Element(queue=w215, element=w217, error in (no error)=w213) -> (error out=w214:errorcluster)  [unwired: 1 in, 2 out]
      }
    }
    n141 = property on="Node Info" class="Clust (strict)"(error in=w198, "Value"=w202) -> ()  [unwired: 1 in, 2 out]
    n142 = property on="Sensors" class="Clust (strict)"(error in=w198, "Value"=w201) -> ()  [unwired: 1 in, 2 out]
    n143 = flat-sequence {
      tunnel: [w219] -> w197
      tunnel: w198 -> [w219]
      frame #0 {
        n144 = Wait (ms)(milliseconds to wait=u32 100) -> ()  [unwired: 1 out]
      }
    }
  }
  n145 = while {
    tunnel: w10 -> [w399]
    tunnel: w9 -> [w404]
    tunnel: [w401] -> w3
    tunnel: w4 -> [w398]
    stop <- w403 stop-if-true
    # "Producer Loop"
    n146 = event shown="[3] \"gRPC Connect\": Value Change" {
      selector: w398 -> [_ _ _ _ _ _ _ w449]
      dyn-events: _ -> [_ _ _ _ _ _ _ _]
      timeout: _ -> [_ _ _ _ _ _ _ _]
      tunnel: w399 -> [_ w407 w414 w420 w427 w433 w440 w447]
      tunnel: w404 -> [w405 w408 w415 w421 w428 w434 w441 w446]
      tunnel: [w405 w409 w416 w422 w429 w435 w439 w448] -> w401
      tunnel: [_ _ _ _ _ _ _ TRUE ("Stop")] -> w402
      event Timeout {
        n147 = event-data() -> ()  [unwired: 1 in, 3 out]
      }
      event Value Change {
        n148 = event-data() -> ()  [unwired: 1 in, 6 out]
        n149 = Bundle(cluster=T6 {enum."Initialise", variant}, States."gRPC_Update-ValveCtrl", "Control Valves") -> (w410:T6)
        n150 = Enqueue Element(queue=w407, element=w410, error in (no error)=w408) -> (error out=w409:errorcluster)  [unwired: 1 in, 2 out]
      }
      event Value Change {
        n151 = event-data() -> ()  [unwired: 1 in, 6 out]
        n152 = Bundle(cluster=T6 {enum."Initialise", variant}, States."gRPC_Update-PumpCtrl", "Pump Control") -> (w417:T6)
        n153 = Enqueue Element(queue=w414, element=w417, error in (no error)=w415) -> (error out=w416:errorcluster)  [unwired: 1 in, 2 out]
      }
      event "gRPC Connect": Value Change {
        n154 = event-data() -> ()  [unwired: 1 in, 6 out]
        n155 = Bundle(cluster=T6 {enum."Initialise", variant}, States."gRPC_Connect") -> (w423:T6)  [unwired: 1 in]
        n156 = Enqueue Element(queue=w420, element=w423, error in (no error)=w421) -> (error out=w422:errorcluster)  [unwired: 1 in, 2 out]
      }
      event "Server Address": Value Change {
        n157 = event-data() -> ()  [unwired: 1 in, 6 out]
        n158 = Bundle(cluster=T6 {enum."Initialise", variant}, States."Update Settings", "Server Address") -> (w430:T6)
        n159 = Enqueue Element(queue=w427, element=w430, error in (no error)=w428) -> (error out=w429:errorcluster)  [unwired: 1 in, 2 out]
      }
      event "gRPC Disconnect": Value Change {
        n160 = event-data() -> ()  [unwired: 1 in, 6 out]
        n161 = Bundle(cluster=T6 {enum."Initialise", variant}, States."gRPC_Disconnect") -> (w436:T6)  [unwired: 1 in]
        n162 = Enqueue Element(queue=w433, element=w436, error in (no error)=w434) -> (error out=w435:errorcluster)  [unwired: 1 in, 2 out]
      }
      event "Stop": Value Change {
        n163 = event-data() -> ()  [unwired: 1 in, 6 out]
        n164 = Bundle(cluster=T6 {enum."Initialise", variant}, States."Stop") -> (w442:T6)  [unwired: 1 in]
        n165 = Enqueue Element(queue=w440, element=w442, error in (no error)=w441) -> (error out=w439:errorcluster)  [unwired: 1 in, 2 out]
      }
      event User Event {
        n166 = event-data() -> ()  [unwired: 1 in, 4 out]
        n167 = Release Queue(queue=w447, error in (no error)=w446) -> (error out=w445:errorcluster)  [unwired: 1 in, 2 out]
        n168 = Unregister For Events(event registration refnum=w449, error in=w445) -> (error out=w448:errorcluster)
      }
    }
    n169 = Unbundle By Name(w401) -> ("status"=w400:bool)
    n170 = Or(x=w400, y=w402) -> (x .or. y?=w403:bool)
  }
  n171 = Destroy User Event(user event=w1, error in=w3) -> (error out=w2:errorcluster)
  n172 = Merge Errors(w18, w2) -> (w17:errorcluster)
  n173 = call <vilib>:"Simple Error Handler.vi"("error in (no error)"=w17) -> ("error out"=w16:errorcluster)  [unwired: 4 in, 4 out]
  n174 = call <vilib>:"Clear Errors.vi"("error in (no error)"=w16) -> ("error out"=→"Error":errorcluster)  [unwired: 5 in, 1 out]
